vi "JSOn Object Probe.vi"(11 "JSON Value.lvclass":refnum<class "JSON Value.lvclass">) -> (2 "Value String":string, 3 "Boolean":bool)   [LabVIEW 2011, in "JSON Value.lvclass"]
uses:
  JSON Value.lvclass
panel:
  out "JSON Pretty String":string
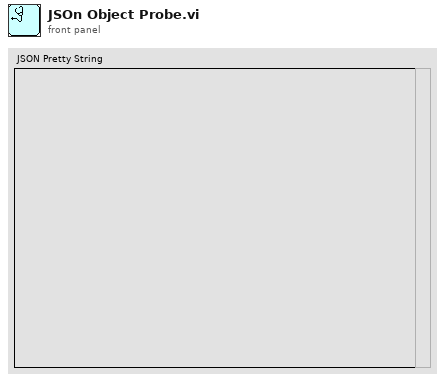
[diagram p1: front panel]
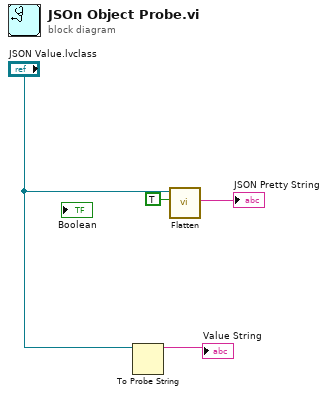
[diagram p0: block diagram]
diagram:
  n1 = To Probe String(7:"JSON Value.lvclass") -> (3:→"Value String":string)  [unwired: 2 in, 1 out]
  n2 = call-dynamic "Flatten.vi"("Pretty Print?"=TRUE, "JSON Value in"="JSON Value.lvclass") -> ("String"=→"JSON Pretty String":string)  [unwired: 8 in, 1 out]
